vi "Conversion.vi"(8 "error in (no error)":errorcluster, 10 "Sensor Type":T3, 11 "Analog Channels":cluster{u16, u16, u16, u16, u16, u16}) -> (0 "error out":errorcluster, 3 "Converted Values":T1)   [LabVIEW 2015]
uses:
  Sensor.ctl
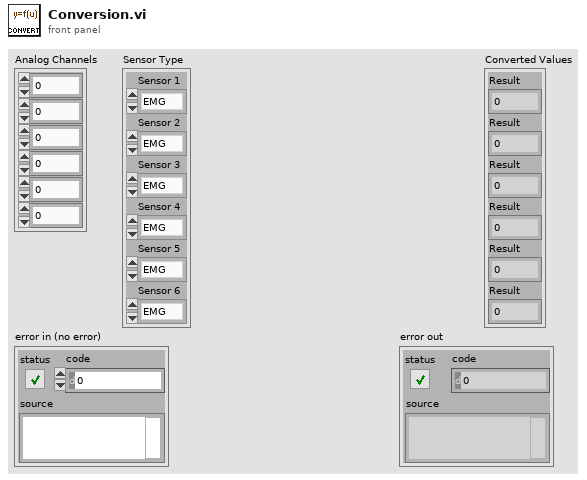
[diagram p1: front panel]
types:
  T1 = cluster{"Result":dbl, "Result":dbl, "Result":dbl, "Result":dbl, "Result":dbl, "Result":dbl}
  T2 = typedef "Sensor.ctl" = enum16{"EMG", "ECG", "EEG", "EDA", "ACC", "LUX"}
  T3 = cluster{"Sensor 1":T2, "Sensor 2":T2, "Sensor 3":T2, "Sensor 4":T2, "Sensor 5":T2, "Sensor 6":T2}
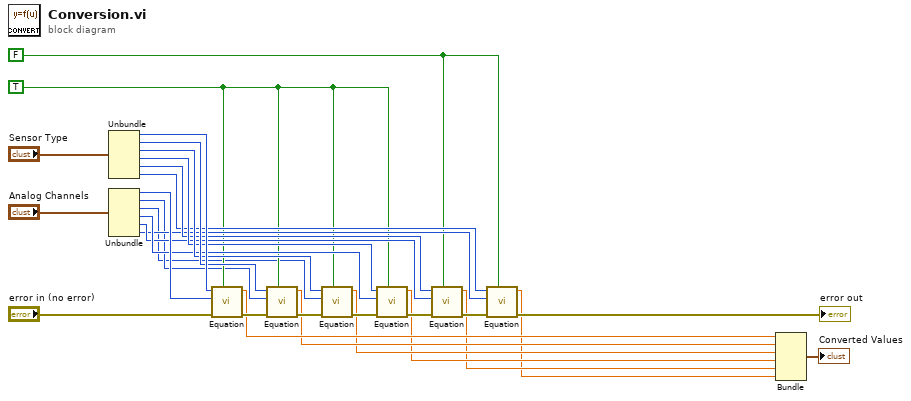
[diagram p0: block diagram]
diagram:
  w19 = FALSE ("10bit")
  w20 = TRUE
  n1 = Unbundle("Sensor Type") -> ("Sensor 1"=w30:T2, "Sensor 2"=w28:T2, "Sensor 3"=w27:T2, "Sensor 4"=w26:T2, "Sensor 5"=w24:T2, "Sensor 6"=w22:T2)
  n2 = Unbundle("Analog Channels") -> (w29:u16, w4:u16, w3:u16, w25:u16, w23:u16, w21:u16)
  n3 = call "Equation.vi"("10bit"=w20, "error in (no error)"="error in (no error)", "Value"=w29, "Sensor Type"=w30) -> ("error out"=w18:errorcluster, "Result"=w10:dbl)  [unwired: 6 in]
  n4 = call "Equation.vi"("10bit"=w20, "error in (no error)"=w18, "Value"=w4, "Sensor Type"=w28) -> ("error out"=w17:errorcluster, "Result"=w9:dbl)  [unwired: 6 in]
  n5 = call "Equation.vi"("10bit"=w20, "error in (no error)"=w17, "Value"=w3, "Sensor Type"=w27) -> ("error out"=w16:errorcluster, "Result"=w8:dbl)  [unwired: 6 in]
  n6 = call "Equation.vi"("10bit"=w20, "error in (no error)"=w16, "Value"=w25, "Sensor Type"=w26) -> ("error out"=w15:errorcluster, "Result"=w7:dbl)  [unwired: 6 in]
  n7 = call "Equation.vi"("10bit"=w19, "error in (no error)"=w15, "Value"=w23, "Sensor Type"=w24) -> ("error out"=w14:errorcluster, "Result"=w6:dbl)  [unwired: 6 in]
  n8 = call "Equation.vi"("10bit"=w19, "error in (no error)"=w14, "Value"=w21, "Sensor Type"=w22) -> ("error out"=→"error out":errorcluster, "Result"=w5:dbl)  [unwired: 6 in]
  n9 = Bundle("Result"=w10, "Result"=w9, "Result"=w8, "Result"=w7, "Result"=w6, "Result"=w5) -> (→"Converted Values":T1)  [unwired: 1 in]
